vi "AlliGator Decode PI Imaging Metadata.vi"(8 "Error In":errorcluster, 11 "Metadata Text Fields":string[](array[string])) -> (0 "Error Out":errorcluster, 1 "Metadata":T1 {"Date" format="%<%x %.3X>T"}, 3 "Metadata String":string, 4 "bitness":i32, 6 "Correct bit shift":bool)   [LabVIEW 2021, in "AlliGator Files.lvlib"]
doc: "Decodes metadata from a Pi Imaging Gate Image."
uses:
  AlliGator Files.lvlib
  AlliGator RecSettings Metadata.ctl
  5fcfaf13-341d-45d1-b0f7-e971b22d1255.vi
  <vilib>/Comparison/Less/Less Functor/Less Functor.lvclass
panel:
  # "see the AlliGator License on the block diagram (Ctrl+E or Window:Show Block Diagram)"
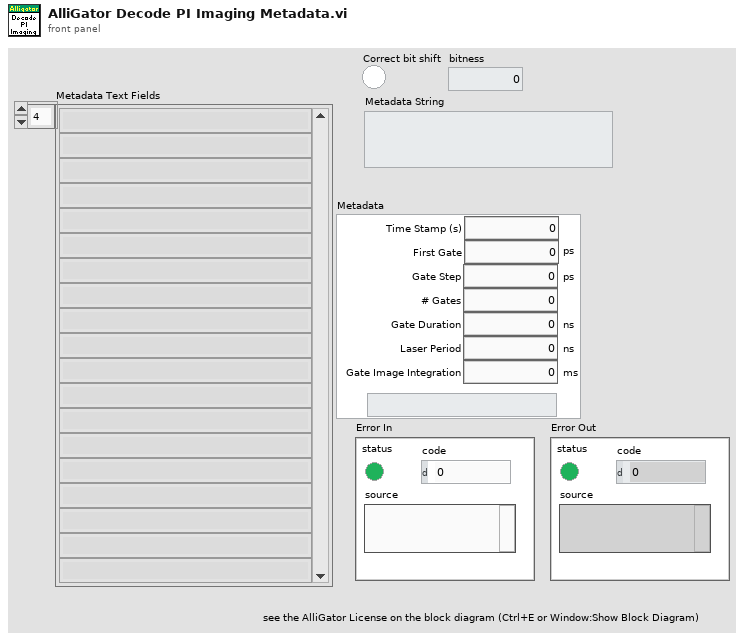
[diagram p1: front panel]
types:
  T1 = typedef "AlliGator Files.lvlib/AlliGator RecSettings Metadata.ctl" = cluster{"Time Stamp (s)":dbl, "First Gate":dbl[unit], "Gate Step":dbl[unit], "# Gates":i32, "Gate Duration":dbl[unit], "Laser Period":dbl[unit], "Gate Image Integration":dbl[unit], "Date":timestamp}
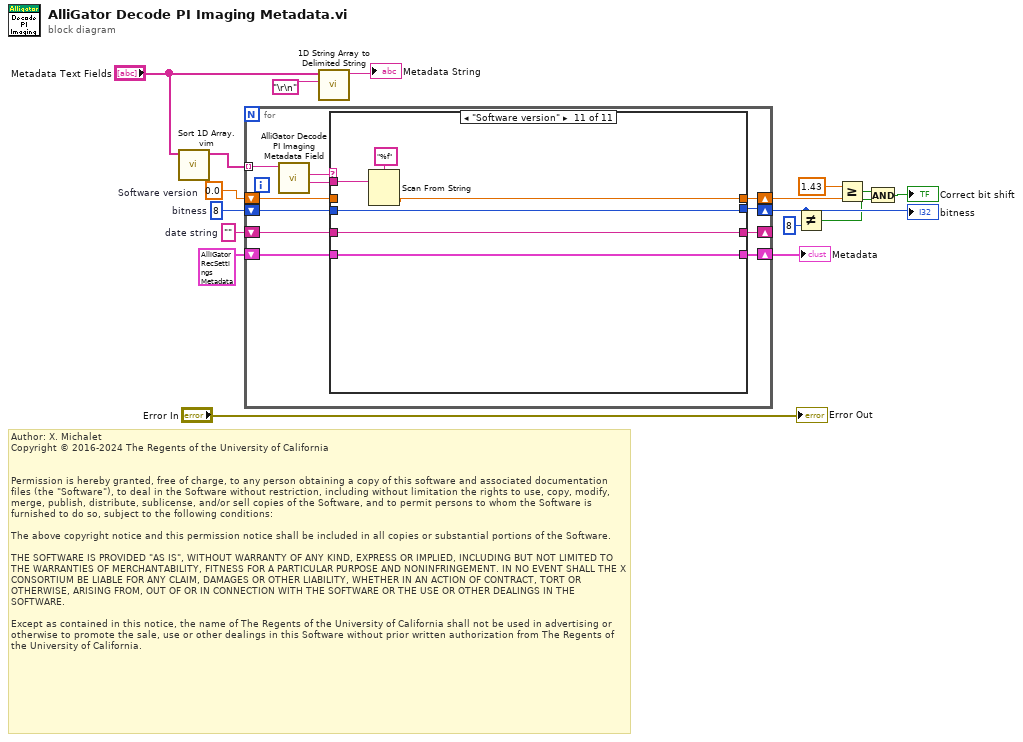
[diagram p0: block diagram]
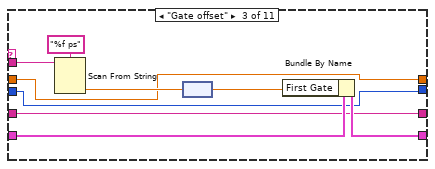
[diagram p4: hidden frame]
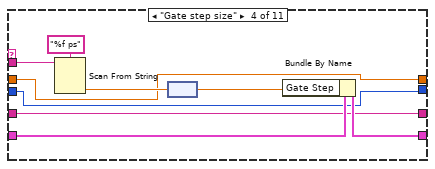
[diagram p5: hidden frame]
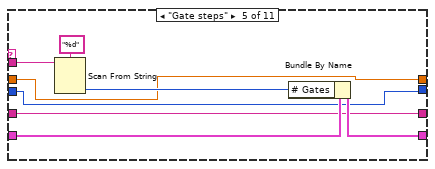
[diagram p6: hidden frame]
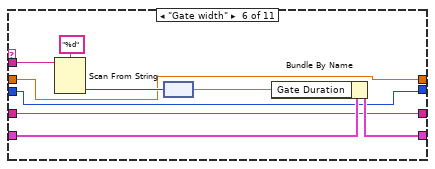
[diagram p7: hidden frame]
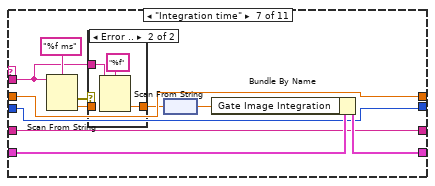
[diagram p8: hidden frame]
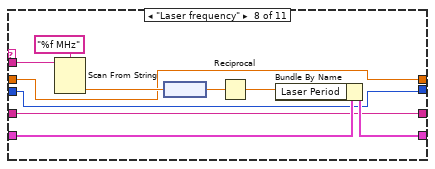
[diagram p10: hidden frame]
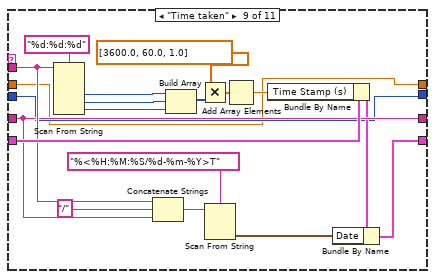
[diagram p11: hidden frame]
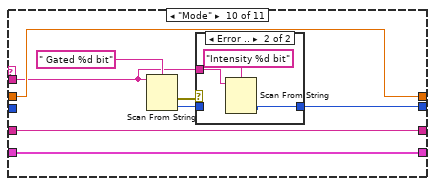
[diagram p12: hidden frame]
diagram:
  w6 = 8  # bitness
  w7 = 0.0  # Software version
  w12 = ""  # date string
  # "Author: X. Michalet\nCopyright © 2016-2024 The Regents of the University of California\n \n\nPermission is hereby granted, free of charge, to any person obtaining a copy of this software and associated documentation files (the \"Software\"), to deal in the Software without restriction, including without limitation the rights to use, copy, modify, merge, publish, distribute, sublicense, and/or sell copies of the Software, and to permit persons to whom the Software is furnished to do so, subject to the following conditions:\n\nThe above copyright notice and this permission notice shall be included in all copies or substantial portions of the Software.\n\nTHE SOFTWARE IS PROVIDED \"AS IS\", WITHOUT WARRANTY OF ANY KIND, EXPRESS OR IMPLIED, INCLUDING BUT NOT LIMITED TO THE WARRANTIES OF MERCHANTABILITY, FITNESS FOR A PARTICULAR PURPOSE AND NONINFRINGEMENT. IN NO EVENT SHALL THE X CONSORTIUM BE LIABLE FOR ANY CLAIM, DAMAGES OR OTHER LIABILITY, WHETHER IN AN ACTION OF CONTRACT, TORT OR OTHERWISE, ARISING FROM, OUT OF OR IN CONNECTION WITH THE SOFTWARE OR THE USE OR OTHER DEALINGS IN THE SOFTWARE.\n\nExcept as contained in this notice, the name of The Regents of the University of California shall not be used in advertising or otherwise to promote the sale, use or other dealings in this Software without prior written authorization from The Regents of the University of California."
  n1 = call "Sort 1D Array.vim"("unsorted array"="Metadata Text Fields") -> ("sorted array"=w13:string[])  [unwired: 10 in]
  n2 = for {
    tunnel: w13 -> [w28] mode=indexing
    shift-right: [w26] -> w10
    shift-left: T1 {"Time Stamp (s)"=0.0, "First Gate"=0.0, "Gate Step"=0.0, "# Gates"=0, "Gate Duration"=0.0, "Laser Period"=0.0, "Gate Image Integration"=0.0, "Date"=timestamp(3757622400 s since 1904-01-01)} ("Metadata") -> [w27]
    shift-right: [w23] -> _
    shift-left: w12 -> [w22]
    shift-right: [w21] -> w9
    shift-left: w6 -> [w20]
    shift-right: [w19] -> w5
    shift-left: w7 -> [w18]
    n3 = call "AlliGator Decode PI Imaging Metadata Field.vi"("Metadata Text Field"=w28) -> ("Metadata"=w25:string, "Field"=w24:string)  [unwired: 9 in]
    n4 = case shown="\"Software version\"" w24 {
      tunnel: w27 -> [w32 w36 w42 w51 w60 w69 w81 w94 w115 w121 w130]
      tunnel: [w32 w36 w40 w49 w58 w67 w80 w92 w99 w121 w130] -> w26
      tunnel: w25 -> [_ w35 w45 w54 w62 w71 w72 w96 w106 w116 w132]
      tunnel: [w31 w35 w39 w48 w57 w65 w78 w89 w104 w123 w133] -> w23
      tunnel: w22 -> [w31 _ w39 w48 w57 w65 w78 w89 w104 w123 w133]
      tunnel: [w30 w34 w38 w47 w56 w64 w77 w88 w98 w117 w129] -> w21
      tunnel: w20 -> [w30 w34 w38 w47 w56 w64 w77 w88 w98 _ w129]
      tunnel: [w29 w33 w37 w46 w55 w63 w76 w87 w97 w120 w128] -> w19
      tunnel: w18 -> [w29 w33 w37 w46 w55 w63 w76 w87 w97 w120 _]
      frame "", Default {
      }
      frame "Date taken" {
      }
      frame "Gate offset" {
        n5 = Scan From String(format string="%f ps", input string=w45) -> (output 1=w43:dbl)  [unwired: 3 in, 3 out]
        n6 = node(w43) -> (w41:dbl[unit])
        n7 = Bundle By Name(cluster=w42, "First Gate"=w41) -> (w40:T1)
      }
      frame "Gate step size" {
        n8 = Scan From String(format string="%f ps", input string=w54) -> (output 1=w52:dbl)  [unwired: 3 in, 3 out]
        n9 = node(w52) -> (w50:dbl[unit])
        n10 = Bundle By Name(cluster=w51, "Gate Step"=w50) -> (w49:T1)
      }
      frame "Gate steps" {
        n11 = Scan From String(format string="%d", input string=w62) -> (output 1=w59:i32)  [unwired: 3 in, 3 out]
        n12 = Bundle By Name(cluster=w60, "# Gates"=w59) -> (w58:T1)
      }
      frame "Gate width" {
        n13 = Scan From String(format string="%d", input string=w71) -> (output 1=w68:i32)  [unwired: 3 in, 3 out]
        n14 = node(w68) -> (w66:dbl[unit])
        n15 = Bundle By Name(cluster=w69, "Gate Duration"=w66) -> (w67:T1)
      }
      frame "Integration time" {
        n16 = Scan From String(format string="%f ms", input string=w72) -> (error out=w75:errorcluster, output 1=w74:dbl)  [unwired: 3 in, 2 out]
        n17 = case shown="Error .." w75 {
          tunnel: w74 -> [w83 _]
          tunnel: [w83 w86] -> w73
          tunnel: w72 -> [_ w84]
          frame No Error {
          }
          frame Error {
            n18 = Scan From String(format string="%f", input string=w84) -> (output 1=w86:dbl)  [unwired: 3 in, 3 out]
          }
        }
        n19 = node(w73) -> (w79:dbl[unit])
        n20 = Bundle By Name(cluster=w81, "Gate Image Integration"=w79) -> (w80:T1)
      }
      frame "Laser frequency" {
        n21 = Scan From String(format string="%f MHz", input string=w96) -> (output 1=w93:dbl)  [unwired: 3 in, 3 out]
        n22 = node(w93) -> (w91:dbl[unit])
        n23 = Reciprocal(x=w91) -> (1/x=w90:dbl[unit])
        n24 = Bundle By Name(cluster=w94, "Laser Period"=w90) -> (w92:T1)
      }
      frame "Time taken" {
        n25 = Scan From String(format string="%d:%d:%d", input string=w106) -> (output 1=w113:i32, output 2=w112:i32, output 3=w111:i32)  [unwired: 5 in, 3 out]
        n26 = Concatenate Strings(w106, "/" ("string"), w104) -> (w105:string)
        n27 = Build Array(w113, w112, w111) -> (w110:i32[])
        n28 = Multiply(x=dbl[] [3600.0, 60.0, 1.0], y=w110) -> (x*y=w108:dbl[])
        n29 = Scan From String(format string="%<%H:%M:%S/%d-%m-%Y>T", input string=w105) -> (output 1=w100:timestamp)  [unwired: 3 in, 3 out]
        n30 = Add Array Elements(numeric array=w108) -> (sum=w107:dbl)
        n31 = Bundle By Name(cluster=w115, "Time Stamp (s)"=w107) -> (w101:T1)
        n32 = Bundle By Name(cluster=w101, "Date"=w100) -> (w99:T1)
      }
      frame "Mode" {
        n33 = Scan From String(format string=" Gated %d bit", input string=w116) -> (error out=w119:errorcluster, output 1=w118:i32)  [unwired: 3 in, 2 out]
        n34 = case shown="Error .." w119 {
          tunnel: w118 -> [w124 _]
          tunnel: [w124 w126] -> w117
          tunnel: w116 -> [_ w125]
          frame No Error {
          }
          frame Error {
            n35 = Scan From String(format string="Intensity %d bit", input string=w125) -> (output 1=w126:i32)  [unwired: 3 in, 3 out]
          }
        }
      }
      frame "Software version" {
        n36 = Scan From String(format string="%f", input string=w132) -> (output 1=w128:dbl)  [unwired: 3 in, 3 out]
      }
    }
  }
  "Metadata" <- w10
  "bitness" <- w9
  n37 = call <vilib>:"1D String Array to Delimited String.vi"("delimiter"="\r\n", "string array"="Metadata Text Fields") -> ("delimited string"=→"Metadata String":string)  [unwired: 9 in]
  n38 = Not Equal?(x=w9, y=8) -> (x != y?=w2:bool)
  n39 = Greater Or Equal?(x=1.43, y=w5) -> (x >= y?=w3:bool)
  n40 = And(x=w3, y=w2) -> (x .and. y?=→"Correct bit shift":bool)
  "Error Out" <- "Error In"
